vi "TestChannels.GetAll.vi"() -> (2 "Channels Paths":T1[](array[typedef]), 3 "Channels Names":string[](array[string]))   [LabVIEW 2015, in "Shared.lvlib"]
uses:
  Shared.lvlib
  Constants.vi
  Channel.Properties.ctl
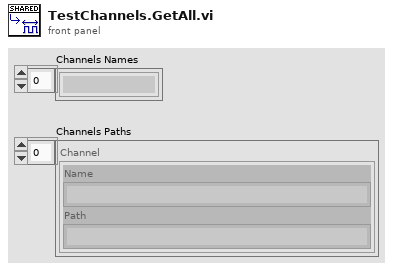
[diagram p1: front panel]
types:
  T1 = typedef "Shared.lvlib/Channel.Properties.ctl" = cluster{"Name":string, "Path":string}
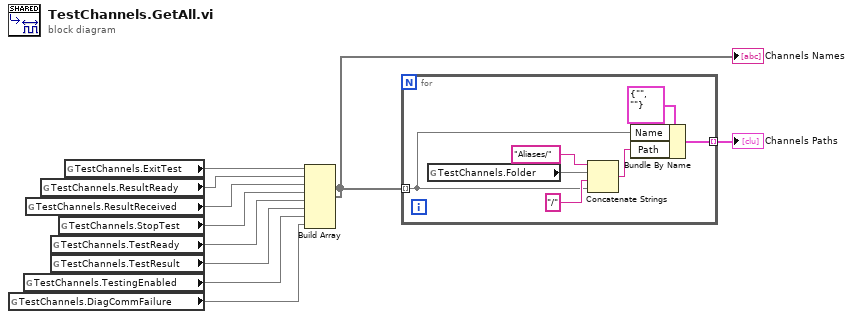
[diagram p0: block diagram]
diagram:
  n1 = global read "Constants.vi" "TestChannels.DiagCommFailure"() -> (w3)
  n2 = global read "Constants.vi" "TestChannels.TestingEnabled"() -> (w4)
  n3 = global read "Constants.vi" "TestChannels.ResultReceived"() -> (w8)
  n4 = global read "Constants.vi" "TestChannels.ResultReady"() -> (w9)
  n5 = global read "Constants.vi" "TestChannels.TestReady"() -> (w6)
  n6 = global read "Constants.vi" "TestChannels.TestResult"() -> (w5)
  n7 = global read "Constants.vi" "TestChannels.StopTest"() -> (w7)
  n8 = global read "Constants.vi" "TestChannels.ExitTest"() -> (w10)
  n9 = Build Array(w10, w9, w8, w7, w6, w5, w4, w3) -> (w1:void[])
  "Channels Names" <- w1
  n10 = for {
    tunnel: w1 -> [w13] mode=indexing
    tunnel: [w11] -> w2 mode=indexing
    n11 = global read "Constants.vi" "TestChannels.Folder"() -> (w17)
    n12 = Concatenate Strings("Aliases/" ("string"), w17, "/" ("string"), w13) -> (w12:string)
    n13 = Bundle By Name(cluster=T1 {"Name"="", "Path"=""}, "Name"=w13, "Path"=w12) -> (w11:T1)
  }
  "Channels Paths" <- w2
